vi "Parse Key and Value.vi"(8 "error in (no error)":errorcluster, 11 "key value pair":string) -> (0 "error out":errorcluster, 1 "Comment":string, 2 "Value":string, 3 "Key":string, 5 "Value_comment":string)   [LabVIEW 2012, in "configlib.lvlib"]
uses:
  configlib.lvlib
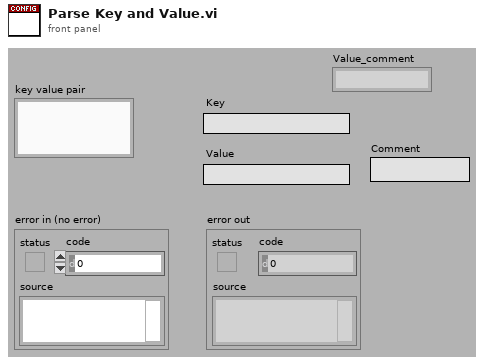
[diagram p1: front panel]
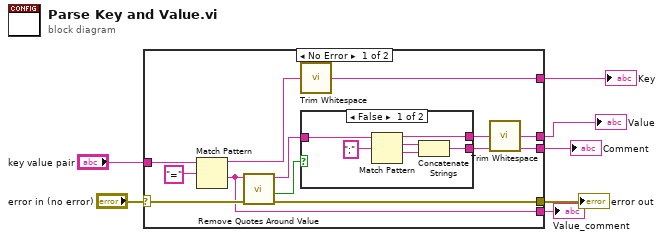
[diagram p0: block diagram]
diagram:
  n1 = case shown="No Error" "error in (no error)" {
    selector: "error in (no error)" -> [w16 w27]
    tunnel: "key value pair" -> [w18 _]
    tunnel: [w15 w27] -> w5
    tunnel: [w14 _] -> w4
    tunnel: [w13 _] -> w3
    tunnel: [w9 _] -> w2
    tunnel: [w8 _] -> w1
    frame No Error {
      n2 = Match Pattern(string=w18, regular expression="=") -> (before substring=w17:string, after substring=w8:string)  [unwired: 1 in, 2 out]
      n3 = call "Remove Quotes Around Value.vi"("error in (no error)"=w16, "string"=w8) -> ("error out"=w15:errorcluster, "in quotes?"=w12:bool, "without quotes"=w10:string)  [unwired: 7 in]
      n4 = call <vilib>:"Trim Whitespace.vi"("string"=w17) -> ("trimmed string"=w14:string)  [unwired: 1 in]
      n5 = case shown="False" w12 {
        tunnel: [w23 w26] -> w11
        tunnel: w10 -> [w24 w26]
        tunnel: [w20 _] -> w9
        frame False {
          n6 = Match Pattern(string=w24, regular expression=";") -> (before substring=w23:string, match substring=w22:string, after substring=w21:string)  [unwired: 1 in, 1 out]
          n7 = Concatenate Strings(w22, w21) -> (w20:string)
        }
        frame True {
        }
      }
      n8 = call <vilib>:"Trim Whitespace.vi"("string"=w11) -> ("trimmed string"=w13:string)  [unwired: 1 in]
    }
    frame Error {
    }
  }
  "error out" <- w5
  "Key" <- w4
  "Value" <- w3
  "Comment" <- w2
  "Value_comment" <- w1
